vi "cluster_v07.vi"() -> ()   [LabVIEW 2009]
panel:
  out "alfa":dbl=6.283185307179558
  in  "stop":bool
  in  "n":u8(slide)=4 scale=0.0..10.0
  out "Roza polara":cluster{dbl[], dbl[]}(graph) caption="XY Graph"
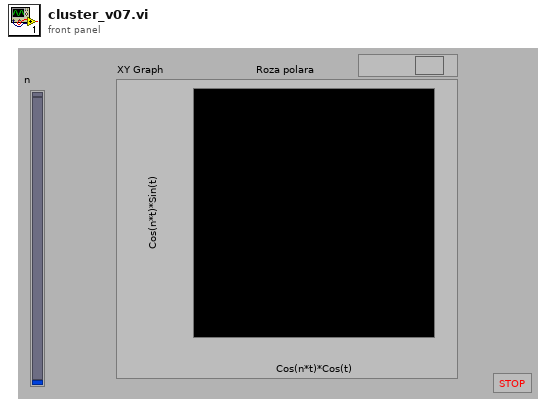
[diagram p1: front panel]
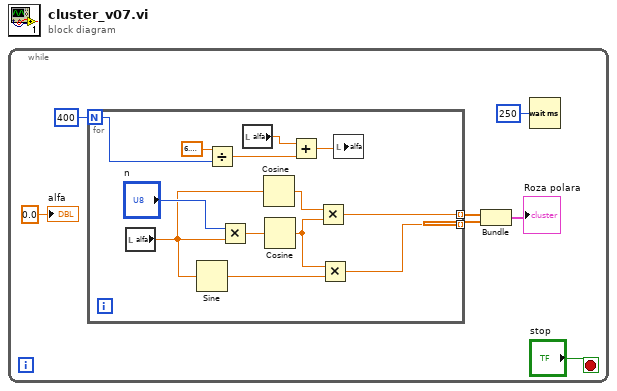
[diagram p0: block diagram]
diagram:
  n1 = while {
    stop <- "stop" stop-if-true
    n2 = for {
      N: 400 -> [w9]
      tunnel: [w18] -> w6 mode=indexing
      tunnel: [w15] -> w5 mode=indexing
      n3 = local read "alfa"() -> (w13:dbl)
      n4 = Sine(x=w13) -> (sin(x)=w16:dbl)
      n5 = Divide(x=6.283185307179586, y=w9) -> (x/y=w10:dbl)
      n6 = Multiply(x="n", y=w13) -> (x*y=w20:dbl)
      n7 = local read "alfa"() -> (w11:dbl)
      n8 = Cosine(x=w13) -> (cos(x)=w19:dbl)
      n9 = Cosine(x=w20) -> (cos(x)=w17:dbl)
      n10 = Add(x=w11, y=w10) -> (x+y=w12:dbl)
      n11 = Multiply(x=w19, y=w17) -> (x*y=w18:dbl)
      n12 = Multiply(x=w17, y=w16) -> (x*y=w15:dbl)
      n13 = local write "alfa"(w12) -> ()
    }
    n14 = Bundle(w6, w5) -> (→"Roza polara":cluster{dbl[], dbl[]})  [unwired: 1 in]
    n15 = Wait (ms)(milliseconds to wait=u32 250) -> ()  [unwired: 1 out]
    "alfa" <- 0.0 ("alfa")
  }
